vi "img.Mean.vi"(9 "IR_img":u16[][](array[numeric])) -> (1 "mean":dbl)   [LabVIEW 2020]
uses:
  <vilib>/Analysis/NI_AALBase.lvlib
  <vilib>/Analysis/baseanly.llb/Mean (DBL).vi
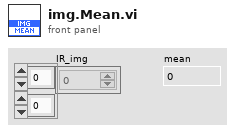
[diagram p1: front panel]
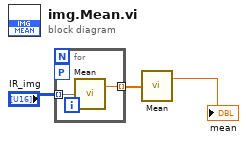
[diagram p0: block diagram]
diagram:
  n1 = for {
    tunnel: "IR_img" -> [w5] mode=indexing
    tunnel: [w4] -> w1 mode=indexing
    workers-P: _ -> [_]
    n2 = call-poly <vilib>:"Mean.vi"("X"=w5) -> ("mean"=w4:dbl)  [unwired: 1 out]
  }
  n3 = call-poly <vilib>:"Mean.vi"("X"=w1) -> ("mean"=→"mean":dbl)  [unwired: 1 out]
